vi "Subvi DO.vi"(2 "DO":refnum<k21>="Connector1/DIO0", 8 "Ext trig enable":bool, 10 "FIFO In":refnum<k21>="DB0") -> ()   [LabVIEW 2017]
uses:
  <vilib>/rvi/Emulation/niFpgaGetClockAttributes.vi
  <vilib>/rvi/Emulation/niFpgaSctlEmulationGetInTimedLoop.vi
  <vilib>/rvi/Emulation/niFpgaEmulationReportErrorSimple.vi
  GV DO delay.vi
  GV FIFO timeout.vi
  <vilib>/rvi/eio/common/nirviEmuTemplateMethod_errors.vi
  <vilib>/rvi/DataTransferAndStorage/Container/Common/niFpgaContainerExecOnDevCompGetState.vi
  <vilib>/rvi/Emulation/niFpgaEmulationIsFPGAContextNoSignature.vi
  <vilib>/rvi/errors/niFpgaSetErrorForExecOnDevCompSimple.vi
  <vilib>/rvi/eio/common/nirviEmuReportErrorAndStop.vi
  <vilib>/rvi/DataTransferAndStorage/Container/Common/niFpgaContainerGetUniqueNameForEmu.vi
  <vilib>/rvi/FIFO/Fifo_Resource/nirvififoEmulationSetSize.vi
  <vilib>/rvi/FIFO/Fifo_Resource/nirviFifoEmulationQueueMgr.vi
  <instcachedir>/0/nirviFifoEmulationQueueMgr_E5CAEC123FF24DC58D834DCA3CDAA9B5.lvgen/nirviFifoEmulationQueueMgr_E5CAEC123FF24DC58D834DCA3CDAA9B5_001.vi
  <vilib>/rvi/FIFO/Fifo_Resource/nirvififoEmulationDetermineInputValidOut.vi
  <vilib>/rvi/FIFO/Fifo_Resource/nirvififoEmulationCreateLock.vi
  <vilib>/rvi/Emulation/niFpgaProcessEmulError.vi
  <vilib>/rvi/FIFO/Fifo_Resource/nirvififoEmulationObtainLock.vi
  <vilib>/rvi/FIFO/Fifo_Resource/nirvififoEmulationReleaseLock.vi
  <vilib>/rvi/occurrence/nirviWaitOnOccurrenceBase.vi
  <vilib>/rvi/errors/nirviReportUnexpectedCaseInternalError.vi
  <vilib>/rvi/errors/nirviReportUnexpectedCaseInternalError (U32).vi
  <vilib>/Utility/error.llb/Clear Errors.vi
  <vilib>/rvi/interface/RandomDataEmulation/niFpgaRandomDataHandleErrors.vi
  <vilib>/rvi/Emulation/niFpgaCriticalErrorInLSC.vi
  <vilib>/eio/EIONode/EIONode.xnode
  <vilib>/rvi/DataTransferAndStorage/Container/XNode/niFpgaContainer.xnode
  <vilib>/rvi/FIFO/Fifo_Resource/niFpgaFifoEmulationRefIn.vi
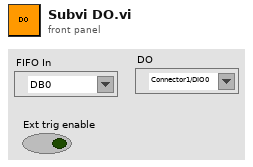
[diagram p1: front panel]
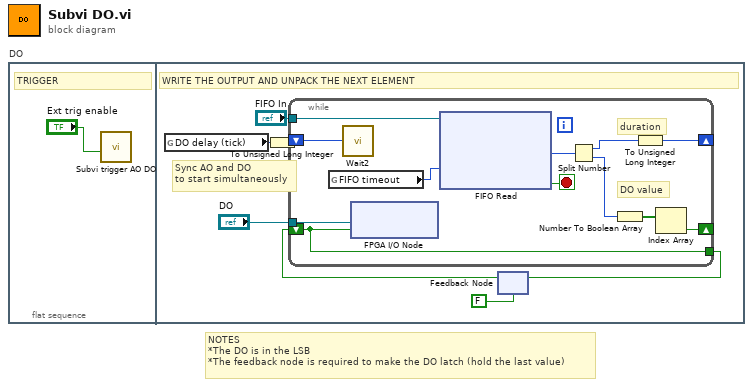
[diagram p0: block diagram]
diagram:
  # "NOTES\n*The DO is in the LSB\n*The feedback node is required to make the DO latch (hold the last value)"
  n1 = flat-sequence "DO" {
    frame #0 {
      # "TRIGGER"
      n2 = call "Subvi trigger AO DO.vi"("Ext trig enable"="Ext trig enable") -> ()  [unwired: 11 in]
    }
    frame #1 {
      # "Sync AO and DO\nto start simultaneously"
      # "WRITE THE OUTPUT AND UNPACK THE NEXT ELEMENT"
      n3 = global read "GV DO delay.vi" "DO delay (tick)"() -> (w4:u16)
      n4 = To Unsigned Long Integer(number=w4) -> (unsigned 32bit integer=w3:u32)
      n5 = feedback #1(FALSE) -> (w7:bool)
      n6 = while {
        shift-right: [w16] -> _
        shift-left: w7 -> [w9]
        shift-right: [w11] -> _
        shift-left: w3 -> [w17]
        tunnel: [w9] -> w6
        tunnel: "FIFO In" -> [w12]
        tunnel: "DO" -> [w10]
        stop <- w14 stop-if-true
        # "DO value"
        # "duration"
        n7 = global read "GV FIFO timeout.vi" "FIFO timeout"() -> (w13:i32)
        n8 = call "Wait2"("Count(Ticks)"=w17) -> ()  [unwired: 1 out]
        n9 = xnode "FPGA I/O Node"("I/O Item"=w9, "FPGA I/O In"=w10) -> ()  [unwired: 1 out]
        n10 = xnode ("FIFO Read")("Timeout"=w13, "FIFO In"=w12) -> ("Element"=w15:u32, "Timed Out?"=w14:bool)  [unwired: 1 out]
        n11 = Split Number(x=w15) -> (hi(x)=w18:u16, lo(x)=w19:u16)
        n12 = Number To Boolean Array(number=w19) -> (Boolean array=w20:bool[])
        n13 = To Unsigned Long Integer(number=w18) -> (unsigned 32bit integer=w11:u32)
        n14 = Index Array(array=w20) -> (element=w16:bool)  [unwired: 1 in]
      }
      n15 = feedback-in #1(w6) -> ()
    }
  }
